vi "Dispenser.vi"(0 "VISA resource name":refnum<visa-resource-name>="COM6", 1 "X":dbl=435.404 format="%#_13g", 3 "Y":dbl=905.746 format="%#_13g", 5 "Serial Configuration":T1={"Baud Rate "=115200, "Parity "=0, "Data Bits "=8, "Stop Bits"=10} {"Stop Bits" items=["1.0"=10, "1.5"=15, "2.0"=20]; "Data Bits" items=["7"=7, "8"=8]; "Parity" items=["None", "Odd", "Even"]; "Baud Rate" items=["9600"=9600, "19200"=19200, "38400"=38400, "115200"=115200]}, 7 "controller in":refnum<k24>, 9 "Path":path=path "C:/Users/TTUHEP/Documents/LabVIEW/Data/Patterns/PCB_base_Dec21_Combined.ngc", 11 "Pressure":dbl[](array[numeric])=[27.0, 27.0, 27.0, 27.0], 12 "Z":dbl=71.609 format="%#_13g", 13 "error in (no error)":errorcluster) -> (4 "Comm":string, 6 "Speed":dbl format="%#_13g", 8 "controller out":refnum<k24>, 10 "Time(ms)":dbl, 15 "error out":errorcluster)   [LabVIEW 2019]
uses:
  C:/Users/TTUHEP/Documents/LabVIEW/Other Models/2010/Bin/Aerotech.A3200.dll
  Other Models/2010/Bin/Aerotech.A3200.dll
  <vilib>/Utility/file.llb/Read Delimited Spreadsheet (string).vi
  Other Models/EFD Ultimus V/EFD Ultimus V.lvlib
panel:
  # "Origin"
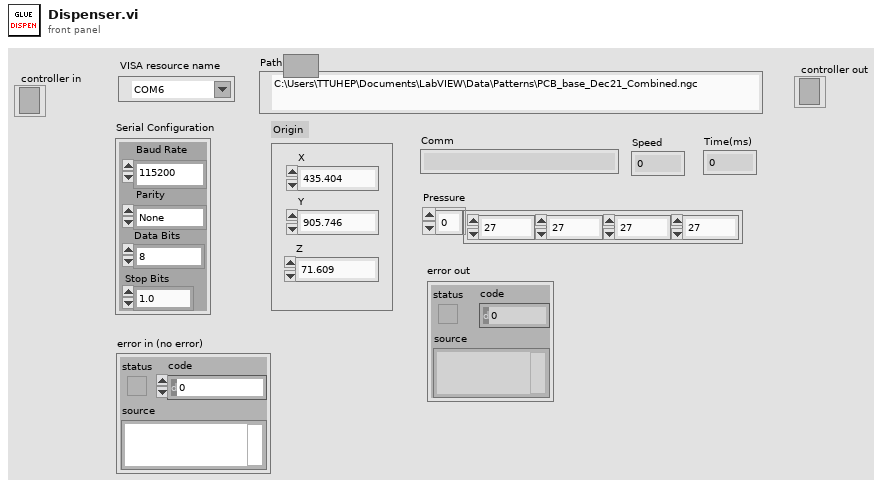
[diagram p1: front panel]
types:
  T1 = cluster{"Baud Rate ":u32, "Parity ":u16, "Data Bits ":u16, "Stop Bits":u16}
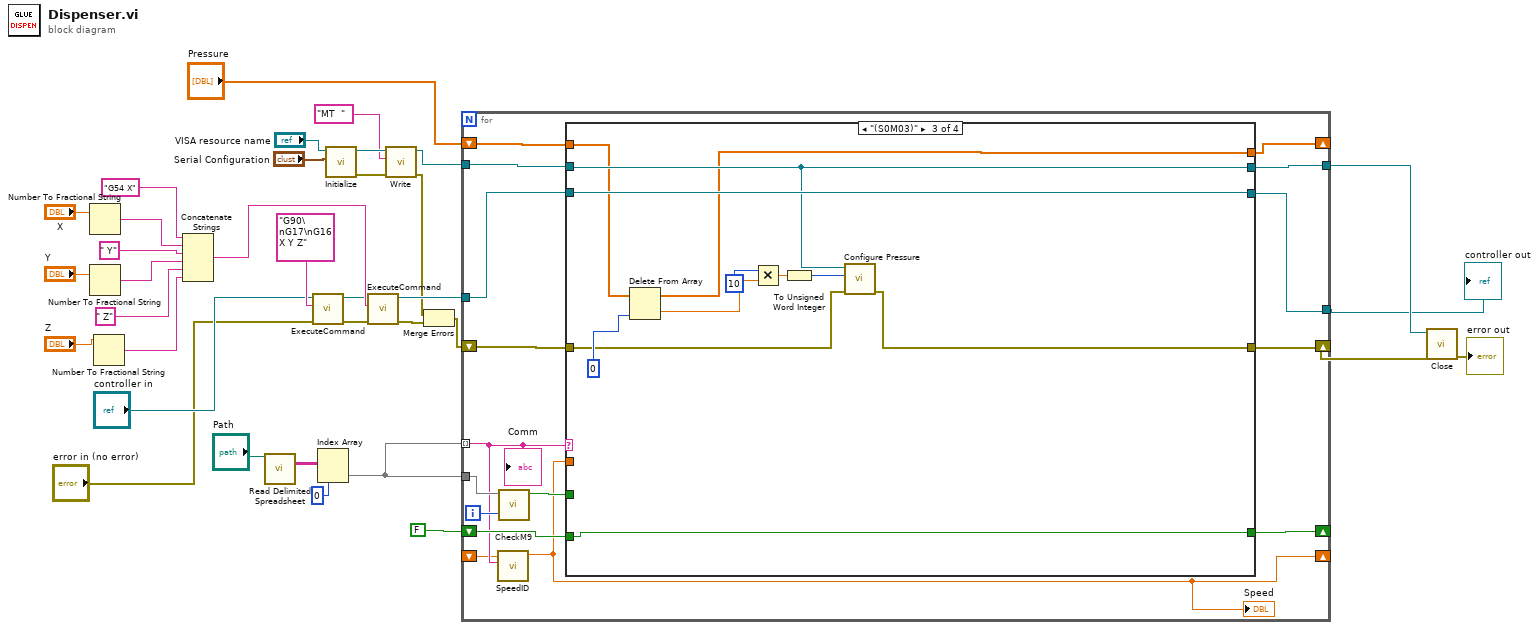
[diagram p0: block diagram]
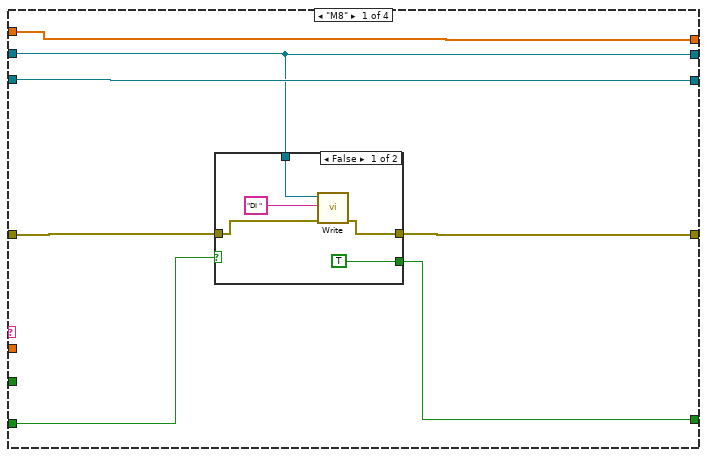
[diagram p2: hidden frame]
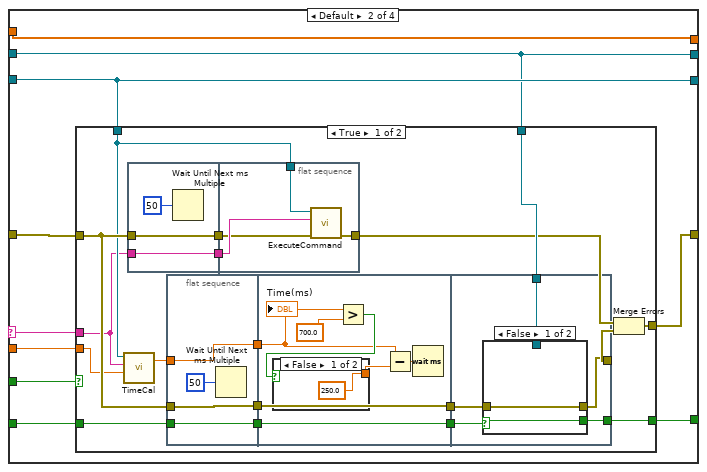
[diagram p4: hidden frame]
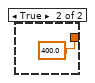
[diagram p5: hidden frame]
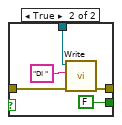
[diagram p6: hidden frame]
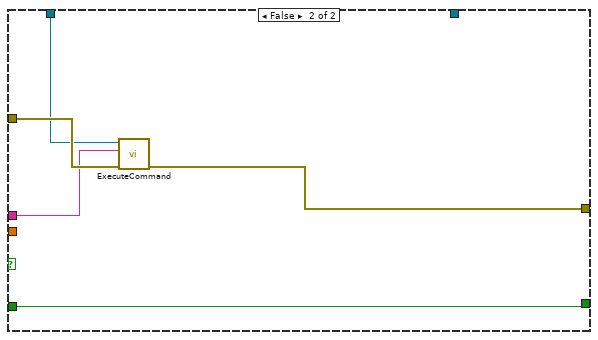
[diagram p7: hidden frame]
diagram:
  n1 = Number To Fractional String(number="X") -> (F-format string=w18:string)  [unwired: 3 in]
  n2 = Number To Fractional String(number="Y") -> (F-format string=w20:string)  [unwired: 3 in]
  n3 = Number To Fractional String(number="Z") -> (F-format string=w22:string)  [unwired: 3 in]
  n4 = Concatenate Strings("G54 X", w18, " Y", w20, " Z", w22) -> (w16:string)
  n5 = call-poly <vilib>:"Read Delimited Spreadsheet.vi"("file path (dialog if empty)"="Path") -> ("all rows"=w34:string[][])  [unwired: 9 in, 5 out]
  n6 = call "ExecuteCommand.vi"("error in (no error)"="error in (no error)", "Command Code"="G90\nG17\nG16 X Y Z", "controller in"="controller in") -> ("error out"=w4:errorcluster, "controller out"=w7:refnum<k24>)  [unwired: 6 in, 1 out]
  n7 = Index Array(array=w34, index (col)=0) -> (element=w9:string[])  [unwired: 1 in]
  n8 = call "Initialize.vi"("Serial Configuration"="Serial Configuration", "VISA resource name"="VISA resource name") -> ("error out"=w13:errorcluster, "VISA resource name out"=w12:refnum<visa-resource-name>)  [unwired: 8 in]
  n9 = call "ExecuteCommand.vi"("error in (no error)"=w4, "Command Code"=w16, "controller in"=w7) -> ("error out"=w28:errorcluster, "controller out"=w31:refnum<k24>)  [unwired: 6 in, 1 out]
  n10 = call "Write.vi"("error in (no error)"=w13, "Command To Write"="MT  ", "VISA resource name"=w12) -> ("error out"=w10:errorcluster, "VISA resource name out"=w14:refnum<visa-resource-name>)  [unwired: 7 in]
  n11 = Merge Errors(w10, w28) -> (w27:errorcluster)
  n12 = for {
    tunnel: w9 -> [w41] mode=indexing
    shift-right: [w38] -> w2
    shift-left: w27 -> [w47]
    shift-right: [w49] -> _
    shift-left: FALSE -> [w50]
    tunnel: w31 -> [w48]
    tunnel: [w51] -> w8
    tunnel: w14 -> [w46]
    tunnel: [w45] -> w26
    tunnel: w9 -> [w44]
    shift-right: [w39] -> _
    shift-left: _ -> [w40]
    shift-right: [w36] -> _
    shift-left: "Pressure" -> [w37]
    i -> [w43]
    n13 = call "SpeedID.vi"("String"=w41, "Speed In"=w40) -> ("Speed Out"=w39:dbl)  [unwired: 9 in]
    "Speed" <- w39
    n14 = call "CheckM9.vi"("Index"=w43, "Comm list"=w44) -> ("Gonna Stop Next"=w42:bool)  [unwired: 9 in]
    n15 = case shown="\"(S0M03)\"" w41 {
      selector: w41 -> [_ w73 _ _]
      tunnel: w47 -> [w53 w75 w132 w146]
      tunnel: w48 -> [w58 w74 w142 w144]
      tunnel: [w57 w67 w131 w146] -> w38
      tunnel: [w58 w74 w142 w144] -> w51
      tunnel: w50 -> [w56 w71 w141 w147]
      tunnel: [w55 w70 w141 w147] -> w49
      tunnel: w46 -> [w54 w72 w140 w145]
      tunnel: [w54 w72 w140 w145] -> w45
      tunnel: w42 -> [_ w69 _ _]
      tunnel: w39 -> [_ w68 _ _]
      tunnel: w37 -> [w52 w66 w138 w143]
      tunnel: [w52 w66 w136 w143] -> w36
      frame "M8" {
        n16 = case shown="False" w56 {
          selector: w56 -> [_ w64]
          tunnel: w53 -> [w61 w65]
          tunnel: [w60 w65] -> w57
          tunnel: [TRUE w64] -> w55
          tunnel: w54 -> [w62 _]
          frame False {
            n17 = call "Write.vi"("error in (no error)"=w61, "Command To Write"="DI ", "VISA resource name"=w62) -> ("error out"=w60:errorcluster)  [unwired: 7 in, 1 out]
          }
          frame True {
          }
        }
      }
      frame Default {
        n18 = case shown="True" w69 {
          tunnel: w75 -> [w85 w130]
          tunnel: [w83 w129] -> w67
          tunnel: w74 -> [w78 w128]
          tunnel: w73 -> [w77 w127]
          tunnel: w72 -> [w91 _]
          tunnel: w71 -> [w93 w126]
          tunnel: [w92 w126] -> w70
          tunnel: w68 -> [w76 _]
          frame True {
            n19 = call "TimeCal.vi"("Speed In"=w76, "Command"=w77, "controller in"=w78) -> ("Time(ms)"=w79:dbl)  [unwired: 7 in, 1 out]
            n20 = flat-sequence {
              tunnel: w77 -> [w120]
              tunnel: [w120] -> w86
              tunnel: w85 -> [w119]
              tunnel: [w119] -> w84
              tunnel: w86 -> [w125]
              tunnel: w84 -> [w124]
              tunnel: [w123] -> w81
              tunnel: w78 -> [w122]
              frame #0 {
                n21 = Wait Until Next ms Multiple(millisecond multiple=50) -> ()  [unwired: 1 out]
              }
              frame #1 {
                n22 = call "ExecuteCommand.vi"("error in (no error)"=w124, "Command Code"=w125, "controller in"=w122) -> ("error out"=w123:errorcluster)  [unwired: 6 in, 2 out]
              }
            }
            n23 = flat-sequence {
              tunnel: w93 -> [w97]
              tunnel: [w97] -> w89
              tunnel: [w95] -> w88
              tunnel: w85 -> [w95]
              tunnel: w79 -> [w94]
              tunnel: [w94] -> w80
              tunnel: [w104] -> w90
              tunnel: w89 -> [w104]
              tunnel: w88 -> [w103]
              tunnel: [w103] -> w87
              tunnel: w80 -> [w98]
              tunnel: [w110] -> w92
              tunnel: [w109] -> w82
              tunnel: w91 -> [w108]
              tunnel: w90 -> [w111]
              tunnel: w87 -> [w107]
              frame #0 {
                n24 = Wait Until Next ms Multiple(millisecond multiple=50) -> ()  [unwired: 1 out]
              }
              frame #1 {
                n25 = Greater?(x=w98, y=700.0) -> (0:w100:bool)
                n26 = case shown="False" w100 {
                  tunnel: [250.0 400.0] -> w101
                  frame False {
                  }
                  frame True {
                  }
                }
                n27 = Subtract(x=w98, y=w101) -> (x-y=w102:dbl)
                n28 = Wait (ms)(milliseconds to wait=w102) -> ()  [unwired: 1 out]
                "Time(ms)" <- w98
              }
              frame #2 {
                n29 = case shown="False" w111 {
                  selector: w111 -> [w112 _]
                  tunnel: w107 -> [w113 w117]
                  tunnel: [w113 w116] -> w109
                  tunnel: [w112 FALSE] -> w110
                  tunnel: w108 -> [_ w115]
                  frame False {
                  }
                  frame True {
                    n30 = call "Write.vi"("error in (no error)"=w117, "Command To Write"="DI ", "VISA resource name"=w115) -> ("error out"=w116:errorcluster)  [unwired: 7 in, 1 out]
                  }
                }
              }
            }
            n31 = Merge Errors(w81, w82) -> (w83:errorcluster)
          }
          frame False {
            n32 = call "ExecuteCommand.vi"("error in (no error)"=w130, "Command Code"=w127, "controller in"=w128) -> ("error out"=w129:errorcluster)  [unwired: 6 in, 2 out]
          }
        }
      }
      frame "(S0M03)" {
        n33 = Delete From Array(array=w138, index=0) -> (deleted portion=w135:dbl, array with subset deleted=w136:dbl[])  [unwired: 1 in]
        n34 = Multiply(x=10, y=w135) -> (x*y=w134:dbl)
        n35 = To Unsigned Word Integer(number=w134) -> (unsigned 16bit integer=w133:u16)
        n36 = call "Configure Pressure.vi"("error in (no error)"=w132, "Pressure Setting (0000)"=w133, "VISA resource name"=w140) -> ("error out"=w131:errorcluster)  [unwired: 7 in, 1 out]
      }
      frame "M9" {
      }
    }
    "Comm" <- w41
  }
  "controller out" <- w8
  n37 = call "Close.vi"("error in (no error)"=w2, "VISA resource name"=w26) -> ("error out"=→"error out":errorcluster)  [unwired: 9 in]
